vi "Save Front panel to Image.vi"(8 "error in (no error)":errorcluster, 10 "FileName":string, 11 "UI_Top_Customer in":refnum<class "UI_Top_Customer.lvclass">) -> (0 "error out":errorcluster, 3 "UI_Top_Customer out":refnum<class "UI_Top_Customer.lvclass">)   [LabVIEW 2021, in "UI_Top_Customer.lvclass"]
uses:
  UI_Top_Customer.lvclass
  UI_Top_Customer.lvclass/UI_Top_Customer.ctl
  <userlib>/John_Lib/TopPath/TopPath.lvlib
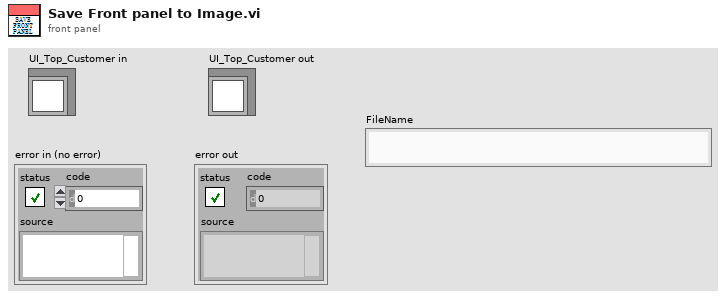
[diagram p1: front panel]
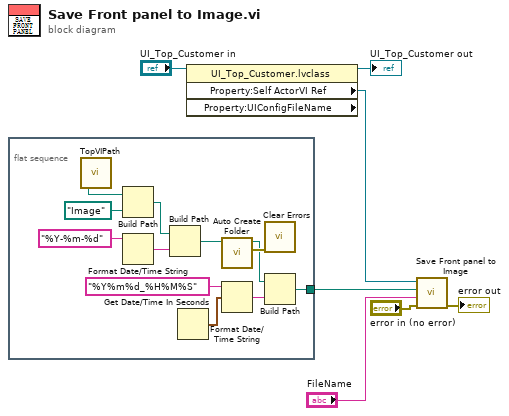
[diagram p0: block diagram]
diagram:
  n1 = flat-sequence {
    tunnel: [w8] -> w3
    frame #0 {
      n2 = call <userlib>:"TopVIPath.vi"() -> ("ResultsData path"=w16:path)  [unwired: 1 in, 2 out]
      n3 = Build Path(base path=w16, name or relative path=path "Image") -> (appended path=w15:path)
      n4 = Format Date/Time String(time format string (%c)="%Y-%m-%d") -> (date/time string=w18:string)  [unwired: 2 in]
      n5 = Build Path(base path=w15, name or relative path=w18) -> (appended path=w14:path)
      n6 = Get Date/Time In Seconds() -> (seconds since 1Jan1904=w12:timestamp)
      n7 = call <userlib>:"Auto Create Folder.vi"("Folder path"=w14) -> ("error out"=w13:errorcluster, "Folder path"=w10:path)  [unwired: 9 in]
      n8 = Format Date/Time String(time format string (%c)="%Y%m%d_%H%M%S", seconds (now)=w12) -> (date/time string=w9:string)  [unwired: 1 in]
      n9 = call <vilib>:"Clear Errors.vi"("error in (no error)"=w13) -> ()  [unwired: 5 in, 2 out]
      n10 = Build Path(base path=w10, name or relative path=w9) -> (appended path=w8:path)
    }
  }
  n11 = property class="UI_Top_Customer.lvclass" props=["Property:Self ActorVI Ref", "Property:UIConfigFileName"](reference="UI_Top_Customer in") -> (reference out=→"UI_Top_Customer out":refnum<class "UI_Top_Customer.lvclass">, "Property:Self ActorVI Ref"=w5:refnum<vi>)  [unwired: 1 in, 2 out]
  n12 = call <userlib>:"Save Front panel to Image.vi"("error in (no error)"="error in (no error)", "FileName"="FileName", "Image Folder Path Include file name"=w3, "vi reference"=w5) -> ("error out"=→"error out":errorcluster)  [unwired: 6 in, 1 out]
